vi "worksheet set default row.vi"(8 "error in (no error)":errorcluster, 9 "hide_unused_rows":u8, 10 "height":dbl, 11 "worksheet":u32) -> (0 "error out":errorcluster)   [LabVIEW 2015, in "xlsxwriter.lvlib"]
doc: "void worksheet_set_default_row(lxw_worksheet worksheet, double height, uint8_t hide_unused_rows);"
uses:
  xlsxwriter.lvlib
  xlsxwriter.dll
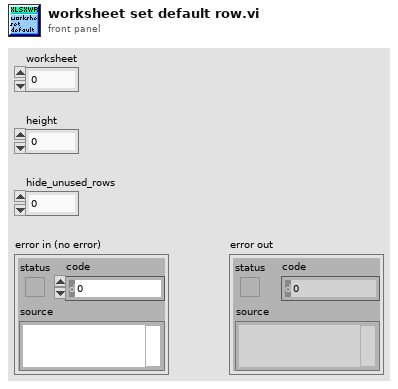
[diagram p1: front panel]
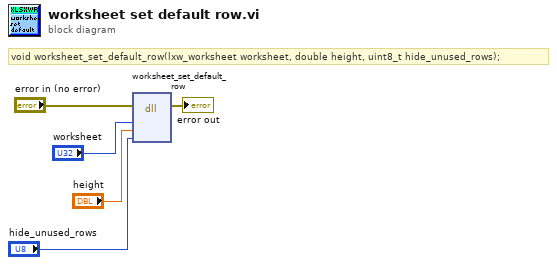
[diagram p0: block diagram]
diagram:
  # "void worksheet_set_default_row(lxw_worksheet worksheet, double height, uint8_t hide_unused_rows);"
  n1 = dll-call lib="C:/Users/WDAGUtilityAccount/Desktop/lv_vis_added_cell/xlsxwriter.*" fn="worksheet_set_default_row"(error in="error in (no error)", "worksheet"="worksheet", "height"="height", "hide_unused_rows"="hide_unused_rows") -> (error out=→"error out":errorcluster)  [unwired: 6 in, 1 out]
